vi "Unify Iterator.vi"(6 "Unified Msgs in":T1, 7 "Actor in":refnum<class "Actor.lvclass">, 9 "Actor Index in":i32=-1, 10 "Actors":refnum<class "Actor.lvclass">[](array[class])) -> (1 "Actor Index out":i32=-1, 4 "Unified Msgs out":T1, 5 "Actor out":refnum<class "Actor.lvclass">)   [LabVIEW 2025, in "jettl.lvlib"]
uses:
  jettl.lvlib
  Actor/Actor.lvclass
  Msgs.ctl
  Msg/Msg.lvclass
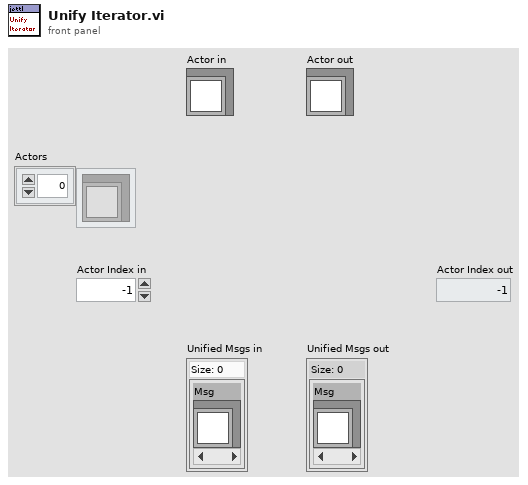
[diagram p1: front panel]
types:
  T1 = typedef "jettl.lvlib/Msgs.ctl" = set{refnum<class "Msg.lvclass">}
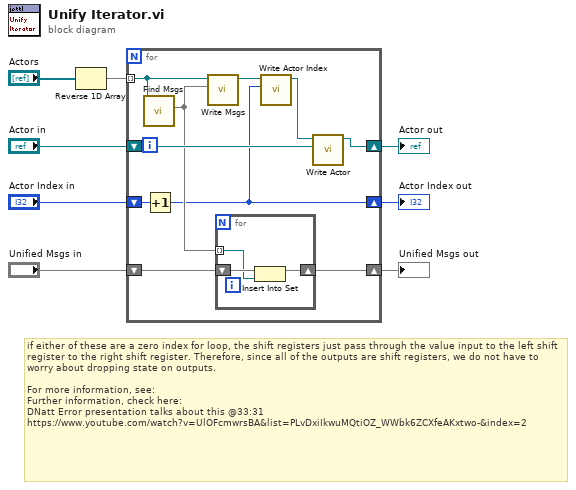
[diagram p0: block diagram]
diagram:
  # "if either of these are a zero index for loop, the shift registers just pass through the value input to the left shift register to the right shift register. Therefore, since all of the outputs are shift registers, we do not have to worry about dropping state on outputs.\n\nFor more information, see:\nFurther information, check here:\nDNatt Error presentation talks about this @33:31\nhttps://www.youtube.com/watch?v=UlOFcmwrsBA&list=PLvDxiIkwuMQtiOZ_WWbk6ZCXfeAKxtwo-&index=2"
  n1 = Reverse 1D Array(array="Actors") -> (reversed array=w8:refnum<class "Actor.lvclass">[])
  n2 = for {
    tunnel: w8 -> [w16] mode=indexing
    shift-right: [w17] -> w7
    shift-left: "Actor in" -> [w18]
    shift-right: [w14] -> w1
    shift-left: "Unified Msgs in" -> [w15]
    shift-right: [w9] -> w4
    shift-left: "Actor Index in" -> [w10]
    n3 = call-dynamic "Find Msgs.vi"("Actor in"=w16) -> ("Msgs"=w13:T1)  [unwired: 10 in]
    n4 = Increment(x=w10) -> (x+1=w9:i32)
    n5 = call-dynamic "Write Msgs.vi"("Msgs"=w13, "Actor in"=w16) -> ("Actor out"=w12:refnum<class "Actor.lvclass">)  [unwired: 9 in]
    n6 = for {
      shift-right: [w20] -> w14
      shift-left: w15 -> [w21]
      tunnel: w13 -> [w19] mode=indexing
      n7 = Insert Into Set(10:w19, 11:w21) -> (3:w20:T1)  [unwired: 1 out]
    }
    n8 = call-dynamic "Write Actor Index.vi"("Actor Index"=w9, "Actor in"=w12) -> ("Actor out"=w11:refnum<class "Actor.lvclass">)  [unwired: 9 in]
    n9 = call-dynamic "Write Actor.vi"("Actor"=w18, "Actor in"=w11) -> ("Actor out"=w17:refnum<class "Actor.lvclass">)  [unwired: 9 in]
  }
  "Actor out" <- w7
  "Unified Msgs out" <- w1
  "Actor Index out" <- w4
